vi "Load Image from File.vi"(8 "error in (no error)":errorcluster, 9 "Image":path, 10 "Load Report":bool, 11 "Launch File Viewer in":refnum<class "Launch File Viewer.lvclass">) -> (0 "error out":errorcluster, 3 "Launch File Viewer out":refnum<class "Launch File Viewer.lvclass">)   [LabVIEW 2014, in "Launch HIJ FileViewer.lvlib" / "Launch File Viewer.lvclass"]
uses:
  Launch File Viewer.lvclass
  HIJ Vision Application/HIJ Vision Application/HIJ Vision Application.lvclass/HIJ Vision Application.ctl
  HIJ Vision File Viewer/HIJ Vision File Viewer Messages/Load Image from File Msg/Load Image from File Msg.lvclass/Load Image from File Msg.ctl
  <vilib>/ActorFramework/Message Enqueuer/Message Enqueuer.lvclass/Message Enqueuer.ctl
  HIJ Vision Application/HIJ Vision Application/Read Display Enq.vi
  <vilib>/ActorFramework/Message Enqueuer/Enqueue.vi
  <vilib>/ActorFramework/Message Priority Queue/Priority Enqueue.vi
  <vilib>/ActorFramework/Message Enqueuer/Message Enqueuer.lvclass
  HIJ Vision File Viewer/HIJ Vision File Viewer Messages/Load Image from File Msg/Load Image from File Msg.lvclass
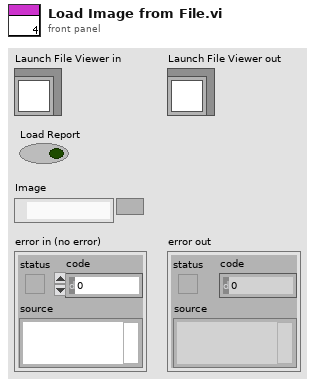
[diagram p1: front panel]
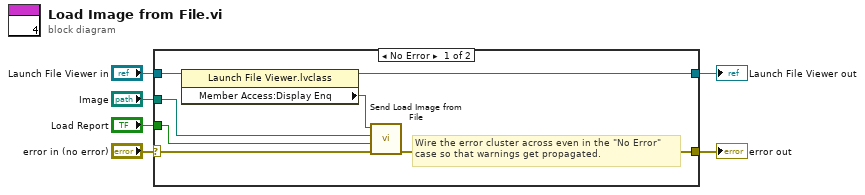
[diagram p0: block diagram]
diagram:
  n1 = case shown="No Error" "error in (no error)" {
    selector: "error in (no error)" -> [w8 w15]
    tunnel: [w7 w15] -> w5
    tunnel: [w12 w14] -> w3
    tunnel: "Launch File Viewer in" -> [w13 w14]
    tunnel: "Load Report" -> [w10 _]
    tunnel: "Image" -> [w9 _]
    frame No Error {
      # "Wire the error cluster across even in the \"No Error\"\ncase so that warnings get propagated."
      n2 = property class="Launch File Viewer.lvclass"(reference=w13) -> (reference out=w12:refnum<class "Launch File Viewer.lvclass">, "Member Access:Display Enq"=w11:refnum<class "Message Enqueuer.lvclass">)  [unwired: 1 in, 1 out]
      n3 = call "Send Load Image from File.vi"("error in (no error)"=w8, "Load Report"=w10, "Path"=w9, "Message Enqueuer"=w11) -> ("error out"=w7:errorcluster)  [unwired: 6 in, 1 out]
    }
    frame Error {
    }
  }
  "error out" <- w5
  "Launch File Viewer out" <- w3
